vi "Simulated VeriStand Engine.Interface.Get Pointers.vi"   [LabVIEW 2016, in "Simulated VeriStand Engine.Interface.lvclass"]
uses:
  Simulated VeriStand Engine.Interface.lvclass
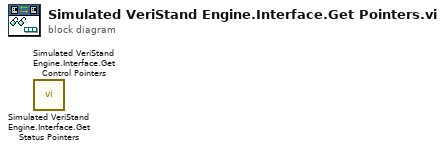
[diagram p0: block diagram]
diagram:
  n1 = call "Simulated VeriStand Engine.Interface.Get Status Pointers.vi"() -> ()  [unwired: 9 in, 3 out]
  n2 = call "Simulated VeriStand Engine.Interface.Get Control Pointers.vi"() -> ()  [unwired: 9 in, 3 out]
